vi "FPGA Main R4 One Loop AB JC KVRev 2.vi"() -> ()   [LabVIEW 2018]
uses:
  <vilib>/eio/EIONode/EIONode.xnode
  <vilib>/rvi/eio/common/nirviEmuTemplateMethod_errors.vi
  Type Defs/Control Mode.ctl
  <vilib>/rvi/Analysis/control/PID/SubVIs/niFpgaPID_PIWrapper.vi
  <vilib>/rvi/DataTransferAndStorage/Container/XNode/niFpgaContainer.xnode
  <vilib>/rvi/interface/RandomDataEmulation/nirviRandomDataFpgaReadWriteTemplate.vi
panel:
  out "Capacitance\nProbe (V) 2":u16
  out "Coil Back \nEMF (V) 2":u16
  in  "Amplifier \nOn/Off 2":bool
  in  "VC Command (V)":u16
  in  "Control Mode":T1=enum."Velocity"
  out "Current Mode":T1=enum."Velocity"
  out "Measuring?":bool
  in  "FFWD/PID":bool
  in  "Amplifier \nOn/Off":bool
  out "Array Index":i32
  out "PID Error (V)":sgl
  out "PID Output (V)":u16
  in  "Output Limits":cluster{"Vmax":sgl, "Vmin":sgl}
  in  "PID Gains":cluster{"Kp":sgl, "Ki":sgl}
  out "Capacitance\nProbe (V)":u16
  out "Coil Back \nEMF (V)":u16
  in  "Loop \nRate (uSec)":u32
  # "Sensors"
  # "Loop Rates"
  # "Controls"
  # "PID Settings"
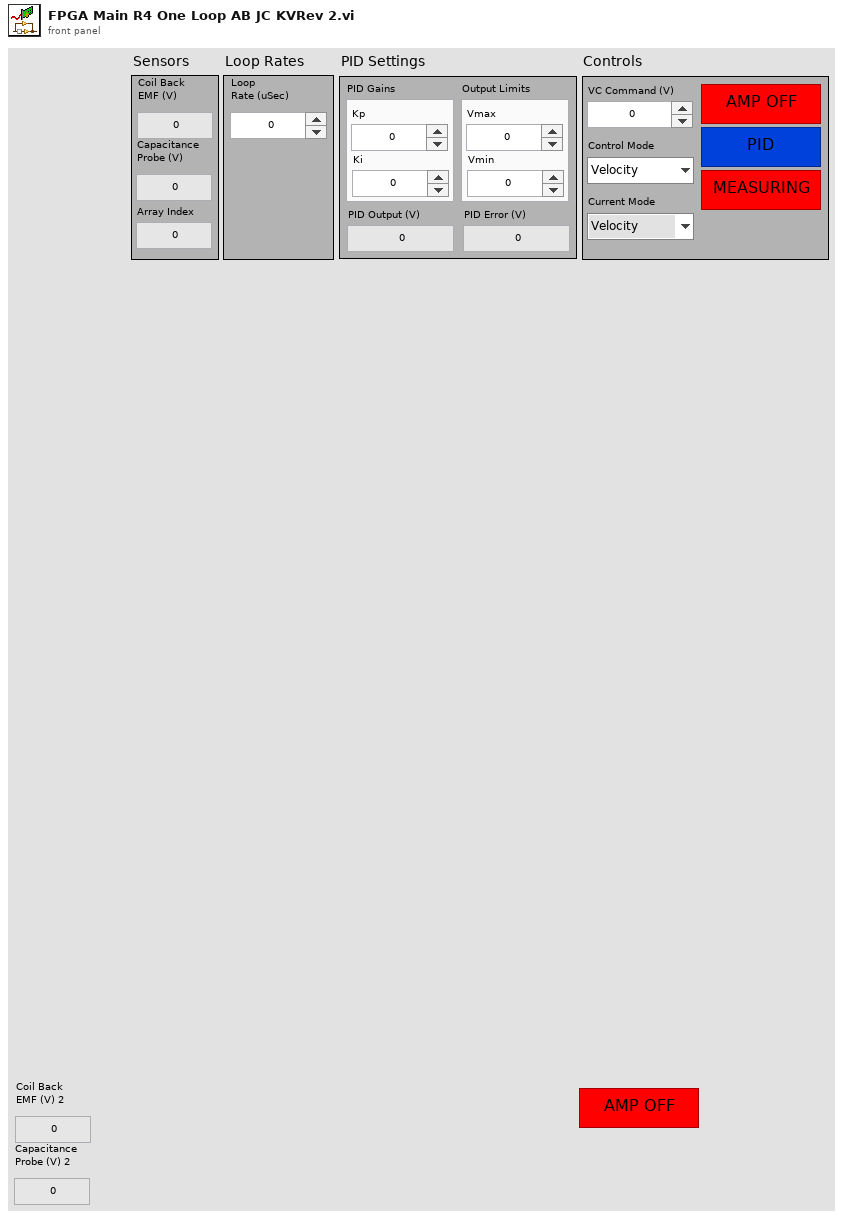
[diagram p1: front panel]
types:
  T1 = typedef "Control Mode.ctl" = enum16{"Start Velocity", "Velocity", "End Velocity", "Displacement", "Manual"}
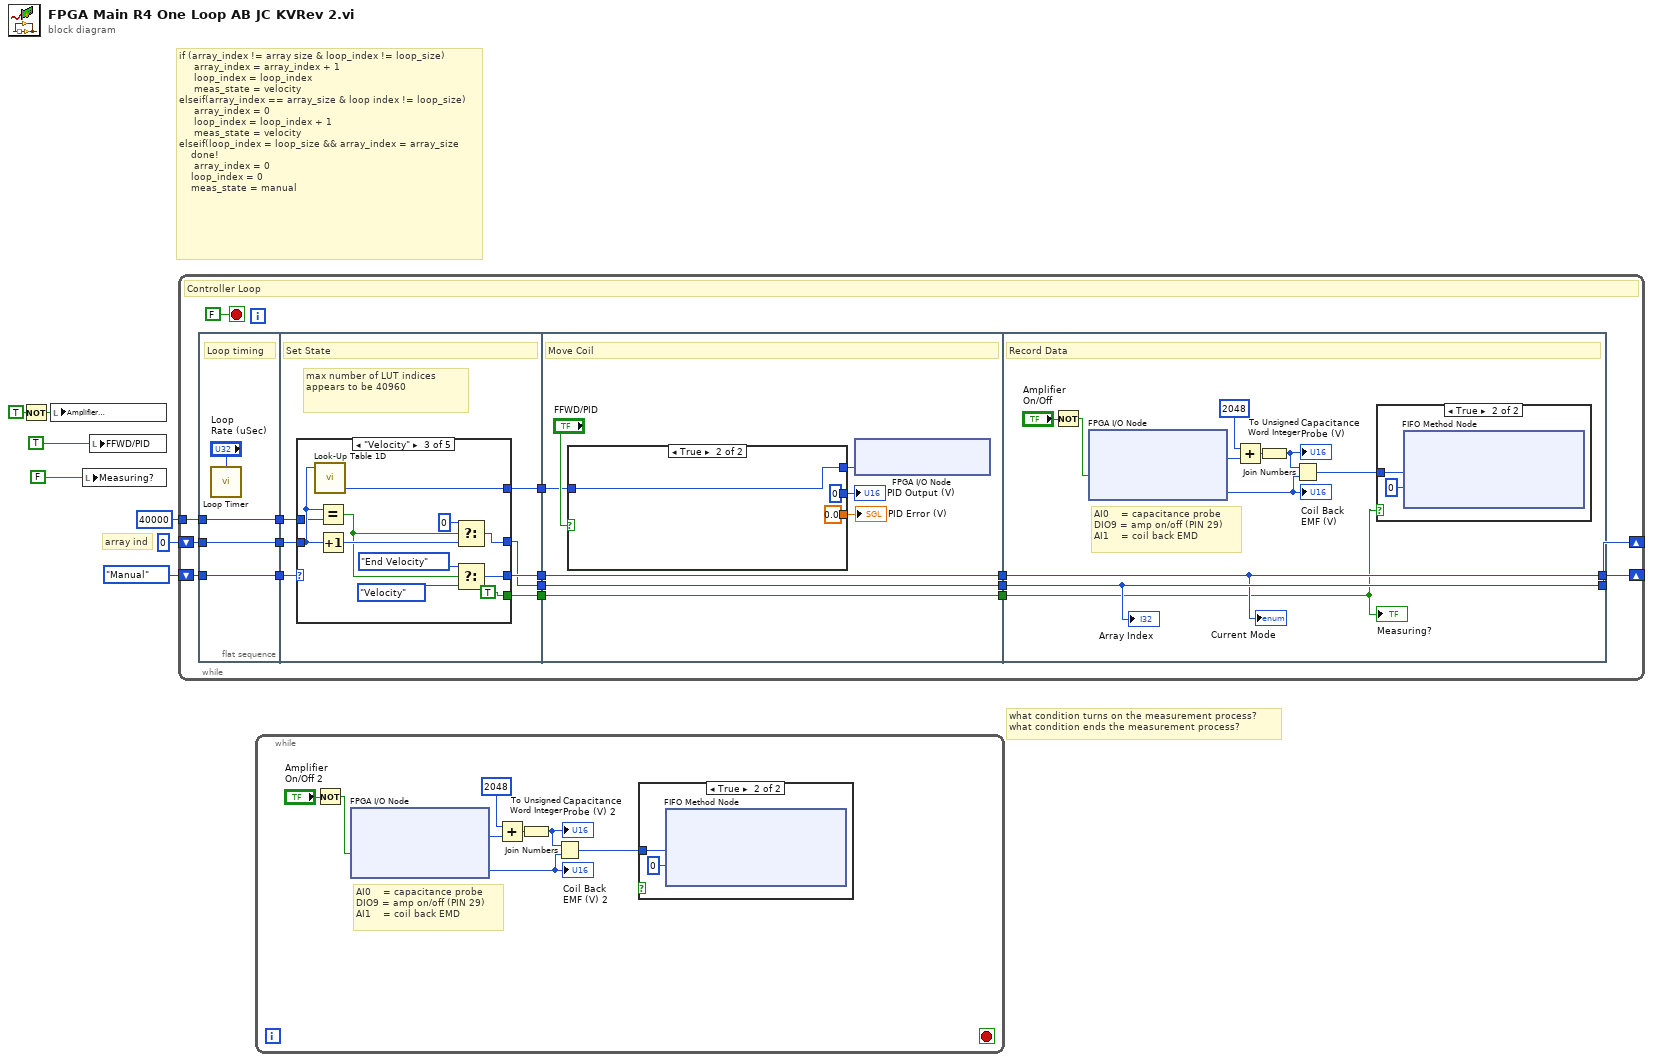
[diagram p0: block diagram]
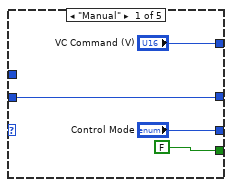
[diagram p3: hidden frame]
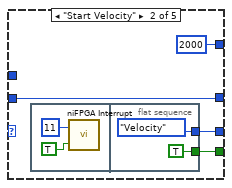
[diagram p4: hidden frame]
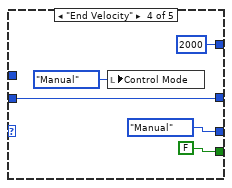
[diagram p5: hidden frame]
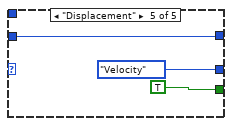
[diagram p6: hidden frame]
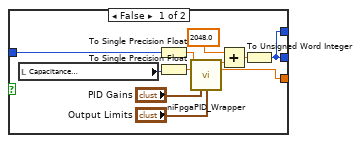
[diagram p7: hidden frame]
diagram:
  # "what condition turns on the measurement process?\nwhat condition ends the measurement process?"
  # "if (array_index != array size & loop_index != loop_size)\n     array_index = array_index + 1\n     loop_index = loop_index\n     meas_state = velocity\nelseif(array_index == array_size & loop index != loop_size)\n     array_index = 0\n     loop_index = loop_index + 1\n     meas_state = velocity\nelseif(loop_index = loop_size && array_index = array_size\n    done!\n     array_index = 0\n    loop_index = 0\n    meas_state = manual"
  # "array ind"
  n1 = Not(x=TRUE) -> (.not. x?=w4:bool)
  n2 = local write "Amplifier \nOn/Off"(w4) -> ()
  n3 = local write "Measuring?"(FALSE) -> ()
  n4 = local write "FFWD/PID"(TRUE) -> ()
  n5 = while {
    shift-right: [w11] -> _
    shift-left: 0 ("index") -> [w22]
    shift-right: [w10] -> _
    shift-left: Control_Mode."Manual" ("Control Mode") -> [w18]
    tunnel: 40000 ("index") -> [w20]
    stop <- FALSE stop-if-true
    # "Controller Loop"
    n6 = flat-sequence {
      tunnel: w22 -> [w26]
      tunnel: [w26] -> w21
      tunnel: w20 -> [w25]
      tunnel: [w25] -> w19
      tunnel: w18 -> [w24]
      tunnel: [w24] -> w17
      tunnel: w21 -> [w34]
      tunnel: w19 -> [w33]
      tunnel: w17 -> [w32]
      tunnel: [w31] -> w16
      tunnel: [w30] -> w15
      tunnel: [w29] -> w14
      tunnel: [w28] -> w9
      tunnel: w16 -> [w69]
      tunnel: w15 -> [w67]
      tunnel: w14 -> [w68]
      tunnel: [w68] -> w13
      tunnel: [w67] -> w12
      tunnel: w9 -> [w66]
      tunnel: [w66] -> w8
      tunnel: w13 -> [w90]
      tunnel: w12 -> [w89]
      tunnel: [w90] -> w11
      tunnel: [w89] -> w10
      tunnel: w8 -> [w88]
      frame #0 {
        # "Loop timing"
        n7 = call "Loop Timer"("Count(uSec)"="Loop \nRate (uSec)") -> ()  [unwired: 1 out]
      }
      frame #1 {
        # "max number of LUT indices appears to be 40960"
        # "Set State"
        n8 = case shown="\"Velocity\"" w32 {
          tunnel: ["VC Command (V)" u16 2000 ("data out") w50 u16 2000 ("data out") _] -> w31
          tunnel: w34 -> [w36 w41 w49 w62 w65]
          tunnel: [w36 w41 w53 w62 w65] -> w29
          tunnel: ["Control Mode" w42 w55 Control_Mode."Manual" ("Control Mode") Control_Mode."Velocity" ("Control Mode")] -> w30
          tunnel: w33 -> [_ _ w48 _ _]
          tunnel: [FALSE w40 TRUE FALSE TRUE] -> w28
          frame "Manual" {
          }
          frame "Start Velocity" {
            n9 = flat-sequence {
              tunnel: [Control_Mode."Velocity" ("Control Mode")] -> w42
              tunnel: [TRUE] -> w40
              frame #0 {
                n10 = call <vilib>:"niFPGA Interrupt.vi"("Wait Until Cleared (F)"=TRUE, "IRQ Number (0)"=u8 11) -> ()  [unwired: 1 in]
              }
              frame #1 {
              }
            }
          }
          frame "Velocity" {
            n11 = call "Look-Up Table 1D"("address"=w49) -> ("data out"=w50:u16)  [unwired: 8 in]
            n12 = Equal?(x=w49, y=w48) -> (x = y?=w51:bool)
            n13 = Increment(x=w49) -> (x+1=w54:i32)
            n14 = Select(t=0 ("index"), s=w51, f=w54) -> (s? t:f=w53:i32)
            n15 = Select(t=Control_Mode."End Velocity" ("Control Mode"), s=w51, f=Control_Mode."Velocity" ("Control Mode")) -> (s? t:f=w55:T1)
          }
          frame "End Velocity" {
            n16 = local write "Control Mode"(Control_Mode."Manual" ("Control Mode")) -> ()
          }
          frame "Displacement" {
          }
        }
      }
      frame #2 {
        # "Move Coil"
        n17 = case shown="True" "FFWD/PID" {
          tunnel: w69 -> [w83 w85]
          tunnel: [w74 u16 0] -> w70
          tunnel: [w77 sgl 0.0 ("error")] -> w71
          tunnel: [w74 w85] -> w73
          frame False {
            n18 = local read "Capacitance\nProbe (V)"() -> (w81:u16)
            n19 = To Single Precision Float(number=w83) -> (single precision float=w82:sgl)
            n20 = To Single Precision Float(number=w81) -> (single precision float=w84:sgl)
            n21 = call-poly <vilib>:"niFpgaPID_Wrapper.vi"("setpoint"=w82, "process variable"=w84, "gains"="PID Gains", "output range"="Output Limits") -> ("output"=w76:sgl, "error"=w77:sgl)  [unwired: 9 in, 1 out]
            n22 = Add(x=sgl 2048.0, y=w76) -> (x+y=w78:sgl)
            n23 = To Unsigned Word Integer(number=w78) -> (unsigned 16bit integer=w74:u16)
          }
          frame True {
          }
        }
        "PID Output (V)" <- w70
        "PID Error (V)" <- w71
        n24 = xnode "FPGA I/O Node"("ConnectorA/AO1"=w73) -> ()  [unwired: 1 in, 1 out]
      }
      frame #3 {
        # "AI0    = capacitance probe\nDIO9 = amp on/off (PIN 29)\nAI1    = coil back EMD"
        # "Record Data"
        n25 = Not(x="Amplifier \nOn/Off") -> (.not. x?=w92:bool)
        n26 = xnode "FPGA I/O Node"("ConnectorA/DIO9"=w92) -> ("ConnectorC/AI0"=w97:i16, "ConnectorA/AI1"=w95:u16)  [unwired: 3 in, 3 out]
        "Coil Back \nEMF (V)" <- w95
        n27 = Add(x=i16 2048, y=w97) -> (x+y=w98:i16)
        n28 = To Unsigned Word Integer(number=w98) -> (unsigned 16bit integer=w94:u16)
        "Capacitance\nProbe (V)" <- w94
        n29 = Join Numbers(hi=w94, lo=w95) -> ((hi.lo)=w96:u32)
        n30 = case shown="True" w88 {
          tunnel: w96 -> [_ w100]
          frame False {
          }
          frame True {
            n31 = xnode ("FIFO Method Node")("Element"=w100, "Timeout"=0) -> ()  [unwired: 1 in, 2 out]
          }
        }
        "Measuring?" <- w88
        "Array Index" <- w90
        "Current Mode" <- w89
      }
    }
  }
  n32 = while {
    stop <- _ stop-if-true
    # "AI0    = capacitance probe\nDIO9 = amp on/off (PIN 29)\nAI1    = coil back EMD"
    n33 = Not(x="Amplifier \nOn/Off 2") -> (.not. x?=w103:bool)
    n34 = xnode "FPGA I/O Node"("ConnectorA/DIO9"=w103) -> ("ConnectorC/AI0"=w108:i16, "ConnectorA/AI1"=w106:u16)  [unwired: 3 in, 3 out]
    "Coil Back \nEMF (V) 2" <- w106
    n35 = Add(x=i16 2048, y=w108) -> (x+y=w109:i16)
    n36 = To Unsigned Word Integer(number=w109) -> (unsigned 16bit integer=w105:u16)
    "Capacitance\nProbe (V) 2" <- w105
    n37 = Join Numbers(hi=w105, lo=w106) -> ((hi.lo)=w107:u32)
    n38 = case shown="True" w101 {
      tunnel: w107 -> [_ w111]
      frame False {
      }
      frame True {
        n39 = xnode ("FIFO Method Node")("Element"=w111, "Timeout"=0) -> ()  [unwired: 1 in, 2 out]
      }
    }
  }
